vi "New Log File Configuration.vi"(8 "error in (no error)":errorcluster, 9 "Default Path":path=path "c:/logs", 10 "Default Name":string="Log File", 11 "Device Ref in":T1=18446744073709551615 format="%.0x") -> (0 "error out":errorcluster, 3 "Device Ref out":T1 format="%.0x")   [LabVIEW 2012, in "Waveform Data Logger System Explorer.lvlib"]
uses:
  Waveform Data Logger System Explorer.lvlib
  <vilib>/NI Veristand/Custom Device API/Custom Device Item Ref.ctl
  <vilib>/NI Veristand/Custom Device API/Custom Device Channel Type.ctl
  <vilib>/NI Veristand/Custom Device API/Custom Device Channel.ctl
  Shared/Types/Start Trigger.ctl
  Shared/Types/Stop Trigger.ctl
  Shared/Classes/Log File Specifications/Log File Specification/File Conflict Operation.ctl
  Shared/Globals/Global GUIDs.vi
  Shared/Globals/Property Strings.vi
  <vilib>/NI Veristand/Custom Device API/Set Item Property (Path).vi
  <vilib>/NI Veristand/Custom Device API/Set Item Property (Boolean).vi
  <vilib>/NI Veristand/Custom Device API/Set Item Property (String).vi
  <vilib>/NI Veristand/Custom Device API/Set Item Property (Double).vi
  <vilib>/NI Veristand/Custom Device API/Set Item Property (U16).vi
  <vilib>/NI VeriStand/Custom Device API/Custom Device API.lvlib
  Shared/Waveform Data Logger Shared.lvlib
  Shared/Classes/Log File Specifications/Log File Specification/Log File Specification.lvclass
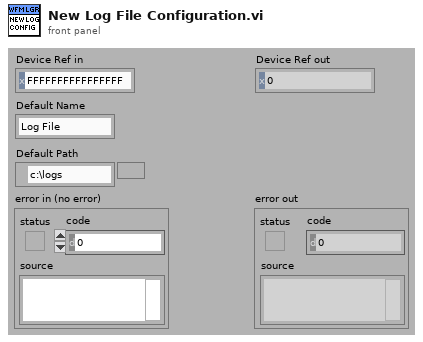
[diagram p1: front panel]
types:
  T1 = typedef "Custom Device API.lvlib/Custom Device Item Ref.ctl" = u64
  T2 = typedef "Waveform Data Logger Shared.lvlib/Log File Specification.lvclass/File Conflict Operation.ctl" = enum16{"Create Unique File Path", "Append to Existing", "Overwrite Existing"}
  T3 = typedef "Waveform Data Logger Shared.lvlib/Stop Trigger.ctl" = enum16{"Log indefinitely", "Stop after duration", "Stop on digital edge", "Stop on analog edge", "Stop when in range", "Stop when out of range", "Stop on value change", "Stop when Boolean condition is true"}
  T4 = typedef "Waveform Data Logger Shared.lvlib/Start Trigger.ctl" = enum16{"Start immediately", "Start on digital edge", "Start on analog edge", "Start when in range", "Start when out of range", "Start on value change", "Start when Boolean condition is true"}
  T5 = typedef "Custom Device API.lvlib/Custom Device Channel Type.ctl" = enum16{"Input", "Output"}
  T6 = typedef "Custom Device API.lvlib/Custom Device Channel.ctl" = cluster{"Type":T5, "Units":string, "Default Value":dbl, "Faultable":bool, "Scalable":bool}
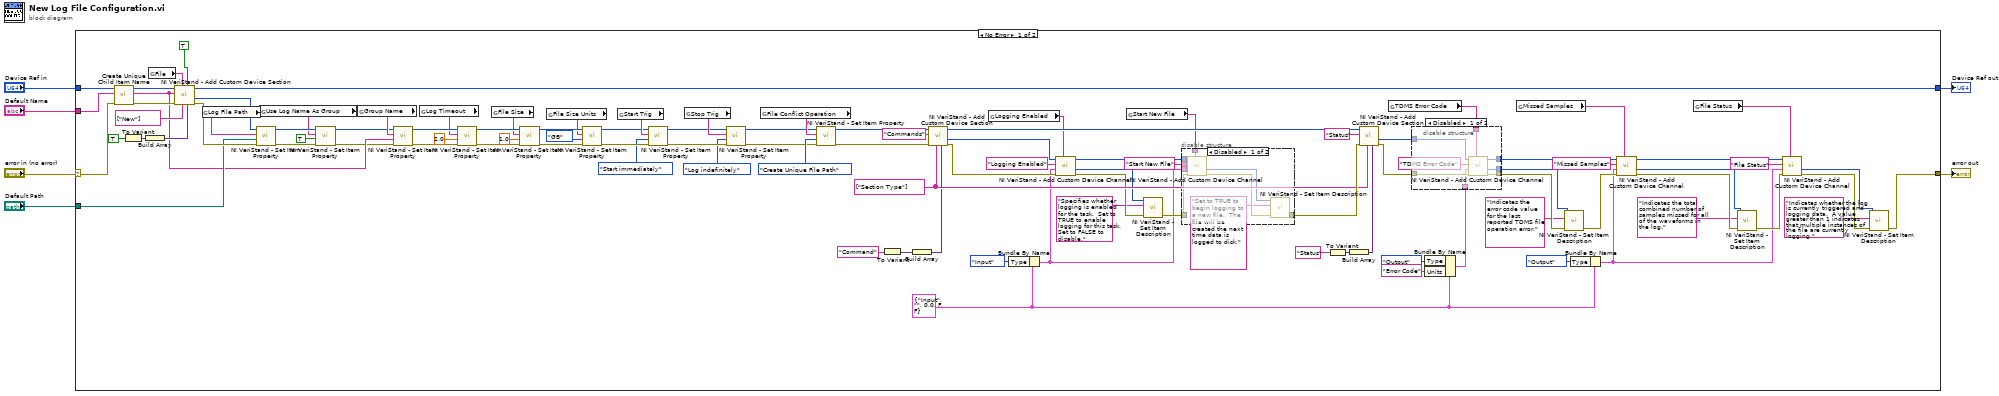
[diagram p0: block diagram]
diagram:
  n1 = case shown="No Error" "error in (no error)" {
    selector: "error in (no error)" -> [w77 w128]
    tunnel: "Default Name" -> [w100 _]
    tunnel: "Default Path" -> [w57 _]
    tunnel: "Device Ref in" -> [w95 w129]
    tunnel: [w94 w129] -> w3
    tunnel: [w13 w128] -> w2
    frame No Error {
      w73 = T6 {"Type"=enum."Input", "Units"="", "Default Value"=0.0, "Faultable"=FALSE, "Scalable"=FALSE} ("Channel")
      w102 = string[] ["Section Type"] ("Property names")
      n2 = call "Create Unique Child Item Name.vi"("error in (no error)"=w77, "Name in"=w100, "Parent Item Ref in"=w95) -> ("error out"=w99:errorcluster, "Unique Name out"=w43:string, "Parent Item Ref out"=w98:T1)  [unwired: 6 out]
      n3 = To Variant(anything=TRUE) -> (Variant=w66:variant)
      n4 = Build Array(w66) -> (w65:variant[])
      n5 = global read "Global GUIDs.vi" "File"() -> (w58:string)
      n6 = call <vilib>:"NI VeriStand - Add Custom Device Section.vi"("Property Values"=w65, "Highlight? (F)"=TRUE, "Property names"=string[] ["New"], "GUID (Default Section)"=w58, "error in (no error)"=w99, "Section Name"=w43, "Parent Ref in"=w98) -> ("error out"=w101:errorcluster, "Section Ptr"=w96:T1, "Parent Ref out"=w94:T1)  [unwired: 2 out]
      n7 = global read "Property Strings.vi" "Log File Path"() -> (w45:string)
      n8 = call-poly <vilib>:"NI VeriStand - Set Item Property.vi"("error in (no error)"=w101, "Value"=w57, "Property Name"=w45, "Item Ref in"=w96) -> ("error out"=w40:errorcluster, "Item Ref out"=w39:T1)  [unwired: 6 out]
      n9 = global read "Property Strings.vi" "Use Log Name As Group"() -> (w38:string)
      n10 = call-poly <vilib>:"NI VeriStand - Set Item Property.vi"("error in (no error)"=w40, "Value"=TRUE ("Default Value"), "Property Name"=w38, "Item Ref in"=w39) -> ("error out"=w41:errorcluster, "Item Ref out"=w42:T1)  [unwired: 6 out]
      n11 = global read "Property Strings.vi" "Group Name"() -> (w44:string)
      n12 = call-poly <vilib>:"NI VeriStand - Set Item Property.vi"("error in (no error)"=w41, "Value"=w43, "Property Name"=w44, "Item Ref in"=w42) -> ("error out"=w35:errorcluster, "Item Ref out"=w36:T1)  [unwired: 6 out]
      n13 = global read "Property Strings.vi" "Log Timeout"() -> (w34:string)
      n14 = call-poly <vilib>:"NI VeriStand - Set Item Property.vi"("error in (no error)"=w35, "Value"=2.0, "Property Name"=w34, "Item Ref in"=w36) -> ("error out"=w31:errorcluster, "Item Ref out"=w32:T1)  [unwired: 6 out]
      n15 = global read "Property Strings.vi" "File Size"() -> (w30:string)
      n16 = call-poly <vilib>:"NI VeriStand - Set Item Property.vi"("error in (no error)"=w31, "Value"=1.0, "Property Name"=w30, "Item Ref in"=w32) -> ("error out"=w27:errorcluster, "Item Ref out"=w28:T1)  [unwired: 6 out]
      n17 = global read "Property Strings.vi" "File Size Units"() -> (w26:string)
      n18 = call-poly <vilib>:"NI VeriStand - Set Item Property.vi"("error in (no error)"=w27, "Value"=enum16{"MB", "GB"}."GB" ("File size units"), "Property Name"=w26, "Item Ref in"=w28) -> ("error out"=w22:errorcluster, "Item Ref out"=w23:T1)  [unwired: 6 out]
      n19 = global read "Property Strings.vi" "Start Trig"() -> (w24:string)
      n20 = call-poly <vilib>:"NI VeriStand - Set Item Property.vi"("error in (no error)"=w22, "Value"=Start_Trigger."Start immediately" ("Value (Signaling)"), "Property Name"=w24, "Item Ref in"=w23) -> ("error out"=w19:errorcluster, "Item Ref out"=w20:T1)  [unwired: 6 out]
      n21 = global read "Property Strings.vi" "Stop Trig"() -> (w21:string)
      n22 = call-poly <vilib>:"NI VeriStand - Set Item Property.vi"("error in (no error)"=w19, "Value"=Stop_Trigger."Log indefinitely" ("Value (Signaling)"), "Property Name"=w21, "Item Ref in"=w20) -> ("error out"=w8:errorcluster, "Item Ref out"=w11:T1)  [unwired: 6 out]
      n23 = global read "Property Strings.vi" "File Conflict Operation"() -> (w12:string)
      n24 = call-poly <vilib>:"NI VeriStand - Set Item Property.vi"("error in (no error)"=w8, "Value"=File_Conflict_Operation."Create Unique File Path" ("File Conflict Operation"), "Property Name"=w12, "Item Ref in"=w11) -> ("error out"=w7:errorcluster, "Item Ref out"=w10:T1)  [unwired: 5 in, 1 out]
      n25 = To Variant(anything="Command" ("String")) -> (Variant=w92:variant)
      n26 = Build Array(w92) -> (w93:variant[])
      n27 = call <vilib>:"NI VeriStand - Add Custom Device Section.vi"("Property Values"=w93, "Property names"=w102, "error in (no error)"=w7, "Section Name"="Commands", "Parent Ref in"=w10) -> ("error out"=w89:errorcluster, "Section Ptr"=w90:T1, "Parent Ref out"=w87:T1)  [unwired: 2 in, 2 out]
      n28 = global read "Global GUIDs.vi" "Logging Enabled"() -> (w47:string)
      n29 = Bundle By Name(cluster=w73, "Type"=Custom_Device_Channel_Type."Input") -> (w48:T6)
      n30 = call <vilib>:"NI VeriStand - Add Custom Device Channel.vi"("GUID (Default Channel)"=w47, "error in (no error)"=w89, "Channel"=w48, "Channel Name"="Logging Enabled", "Parent Ref in"=w90) -> ("error out"=w55:errorcluster, "Channel Ref"=w52:T1, "Parent Ref out"=w49:T1)  [unwired: 3 in, 1 out]
      n31 = global read "Global GUIDs.vi" "Start New File"() -> (w46:string)
      n32 = call <vilib>:"NI VeriStand - Set Item Description.vi"("error in (no error)"=w55, "Description"="Specifies whether logging is enabled for the task.  Set to TRUE to enable logging for this task. Set to FALSE to disable." ("String"), "Item Ref in"=w52) -> ("error out"=w56:errorcluster)  [unwired: 6 in, 2 out]
      n33 = disable-structure shown="Disabled" {
        disable-tunnel: [w125 w127] -> w106
        disable-tunnel: w56 -> [w122 w127]
        disable-tunnel: "Start New File" ("Channel Name") -> [w121 _]
        disable-tunnel: w49 -> [w120 _]
        disable-tunnel: w48 -> [w119 _]
        disable-tunnel: w46 -> [w118 _]
        frame Disabled {
          n34 = call <vilib>:"NI VeriStand - Add Custom Device Channel.vi"("GUID (Default Channel)"=w118, "error in (no error)"=w122, "Channel"=w119, "Channel Name"=w121, "Parent Ref in"=w120) -> ("error out"=w126:errorcluster, "Channel Ref"=w124:T1)  [unwired: 3 in, 2 out]
          n35 = call <vilib>:"NI VeriStand - Set Item Description.vi"("error in (no error)"=w126, "Description"="Set to TRUE to begin logging to a new file.  The file will be created the next time data is logged to disk." ("String"), "Item Ref in"=w124) -> ("error out"=w125:errorcluster)  [unwired: 6 in, 2 out]
        }
        frame Enabled {
        }
      }
      n36 = To Variant(anything="Status" ("String")) -> (Variant=w86:variant)
      n37 = Build Array(w86) -> (w85:variant[])
      n38 = call <vilib>:"NI VeriStand - Add Custom Device Section.vi"("Property Values"=w85, "Property names"=w102, "error in (no error)"=w106, "Section Name"="Status", "Parent Ref in"=w87) -> ("error out"=w83:errorcluster, "Section Ptr"=w84:T1)  [unwired: 2 in, 3 out]
      n39 = global read "Global GUIDs.vi" "TDMS Error Code"() -> (w16:string)
      n40 = Bundle By Name(cluster=w73, "Type"=Custom_Device_Channel_Type."Output", "Units"="Error Code") -> (w80:T6)
      n41 = disable-structure shown="Disabled" {
        disable-tunnel: [w115 w116] -> w105
        disable-tunnel: w84 -> [w113 w117]
        disable-tunnel: w83 -> [w112 w116]
        disable-tunnel: w80 -> [w111 _]
        disable-tunnel: [w110 w117] -> w76
        disable-tunnel: [w109 _] -> w72
        disable-tunnel: w16 -> [w108 _]
        frame Disabled {
          n42 = call <vilib>:"NI VeriStand - Add Custom Device Channel.vi"("GUID (Default Channel)"=w108, "error in (no error)"=w112, "Channel"=w111, "Channel Name"="TDMS Error Code", "Parent Ref in"=w113) -> ("error out"=w115:errorcluster, "Channel Ref"=w109:T1, "Parent Ref out"=w110:T1)  [unwired: 3 in, 1 out]
        }
        frame Enabled {
        }
      }
      n43 = global read "Global GUIDs.vi" "Missed Samples"() -> (w15:string)
      n44 = call <vilib>:"NI VeriStand - Set Item Description.vi"("error in (no error)"=w105, "Description"="Indicates the error code value for the last reported TDMS file operation error." ("String"), "Item Ref in"=w72) -> ("error out"=w103:errorcluster)  [unwired: 6 in, 2 out]
      n45 = Bundle By Name(cluster=w73, "Type"=Custom_Device_Channel_Type."Output") -> (w61:T6)
      n46 = call <vilib>:"NI VeriStand - Add Custom Device Channel.vi"("GUID (Default Channel)"=w15, "error in (no error)"=w103, "Channel"=w61, "Channel Name"="Missed Samples", "Parent Ref in"=w76) -> ("error out"=w104:errorcluster, "Channel Ref"=w70:T1, "Parent Ref out"=w63:T1)  [unwired: 3 in, 1 out]
      n47 = global read "Global GUIDs.vi" "File Status"() -> (w14:string)
      n48 = call <vilib>:"NI VeriStand - Set Item Description.vi"("error in (no error)"=w104, "Description"="Indicates the total combined number of samples missed for all of the waveforms in the log." ("String"), "Item Ref in"=w70) -> ("error out"=w62:errorcluster)  [unwired: 6 in, 2 out]
      n49 = call <vilib>:"NI VeriStand - Add Custom Device Channel.vi"("GUID (Default Channel)"=w14, "error in (no error)"=w62, "Channel"=w61, "Channel Name"="File Status", "Parent Ref in"=w63) -> ("error out"=w107:errorcluster, "Channel Ref"=w59:T1)  [unwired: 3 in, 2 out]
      n50 = call <vilib>:"NI VeriStand - Set Item Description.vi"("error in (no error)"=w107, "Description"="Indicates whether the log is currently triggered and logging data.  A value greater than 1 indicates that multiple instances of the file are currently logging." ("String"), "Item Ref in"=w59) -> ("error out"=w13:errorcluster)  [unwired: 6 in, 2 out]
    }
    frame Error {
    }
  }
  "Device Ref out" <- w3
  "error out" <- w2
